vi "Dan Humidity.vi"() -> ()   [LabVIEW 2012]
uses:
  <vilib>/MakerHub/LINX/LMH-LINX.lvlib
  <vilib>/MakerHub/LINX/Public/Peripherals/Analog/Analog Read 1 Chan.vi
panel:
  out "humidity":dbl(graph)
  in  "Serial Port":refnum<visa-resource-name>="COM7"
  in  "stop":bool
  out "humidity":dbl
  in  "humidity":u8
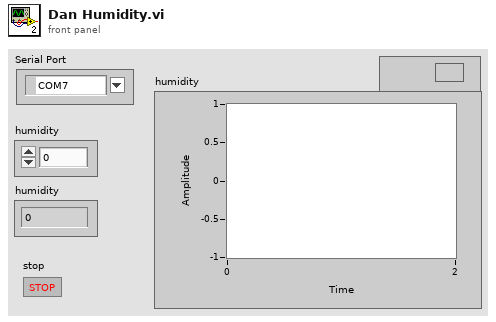
[diagram p1: front panel]
types:
  T1 = typedef "LMH-LINX.lvlib/LINX Ref.ctl" = cluster{"Platform":T2, "Interface":T3, "LINX Device Config":T4}
  T2 = typedef "LMH-LINX.lvlib/Platform.ctl" = enum16{"LINX", "myRIO"}
  T3 = typedef "LMH-LINX.lvlib/Interface.ctl" = enum16{"Serial", "TCP"}
  T4 = typedef "LMH-LINX.lvlib/Device.lvlib/LINX Device Config.ctl" = cluster{"Interface":T3, "COM Port":refnum<visa-resource-name>, "TCP Configuration":T5, "Device Family":u8, "Device ID":u8, "Device Name":string, "TCP Ref":refnum<k5>, "Channels":T6}
  T5 = typedef "LMH-LINX.lvlib/Device.lvlib/TCP Config.ctl" = cluster{"IP Address":string, "Port":u16}
  T6 = typedef "LMH-LINX.lvlib/Channels.ctl" = cluster{"DI":u8[], "DO":u8[], "AI":u8[], "AO":u8[], "PWM":u8[], "QE":u8[], "UART":u8[], "I2C 2":u8[], "SPI":u8[], "CAN":u8[], "Servo":u8[], "AI Ref (V)":dbl, "AO Ref (V)":dbl, "AO Resolution (Bits)":u8}
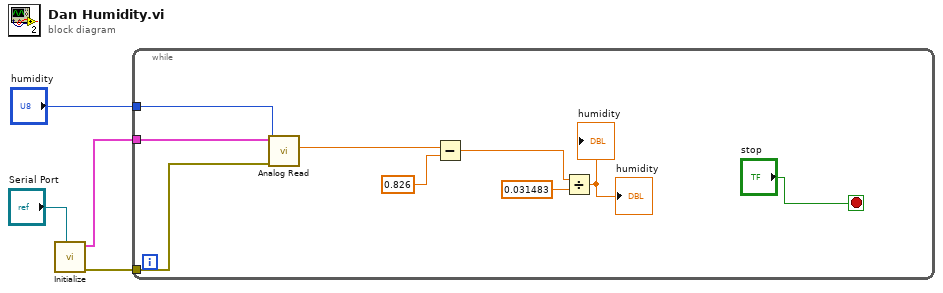
[diagram p0: block diagram]
diagram:
  n1 = call <vilib>:"Initialize.vi"("Serial Port"="Serial Port") -> ("Error Out"=w1:errorcluster, "LINX Ref"=w2:T1)  [unwired: 8 in, 1 out]
  n2 = while {
    tunnel: w2 -> [w13]
    tunnel: w1 -> [w7]
    tunnel: "humidity" -> [w8]
    stop <- "stop" stop-if-true
    n3 = call-poly <vilib>:"Analog Read.vi"("Error In"=w7, "Analog Channel"=w8, "LINX Resource"=w13) -> ("AI Value"=w12:dbl)  [unwired: 5 in, 3 out]
    n4 = Subtract(x=w12, y=0.826) -> (x-y=w10:dbl)
    n5 = Divide(x=w10, y=0.031483) -> (x/y=→"humidity" →"humidity":dbl)
  }
